vi "Set-Test-Clear Saved Tag.vi"(8 "op":enum16{"test", "clear", "set"}(ring), 11 "instVIref":T1) -> (0 "saved":bool, 3 "instVIref out":T1)   [LabVIEW 2020, in "NI_TargetHelper.lvlib"]
uses:
  <vilib>/TargetSupport/NI_TargetHelper/NI_TargetHelper.lvlib
  <vilib>/TargetSupport/NI_TargetHelper/Instance VIref.ctl
  <vilib>/UserTags/UserTags.lvlib
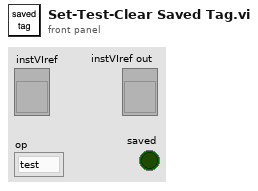
[diagram p1: front panel]
types:
  T1 = typedef "NI_TargetHelper.lvlib/Instance VIref.ctl" = refnum<vi>
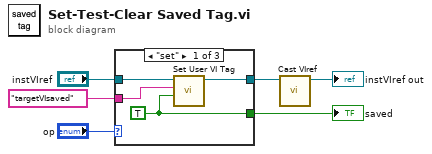
[diagram p0: block diagram]
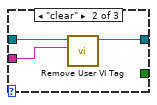
[diagram p2: hidden frame]
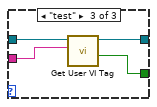
[diagram p3: hidden frame]
diagram:
  n1 = case shown="\"set\"" "op" {
    tunnel: "instVIref" -> [w10 w12 w17]
    tunnel: [w7 _ w14] -> w6
    tunnel: [w9 w11 w16] -> w3
    tunnel: "targetVIsaved" ("Tag Name") -> [w8 w13 w15]
    frame "set" {
      w7 = TRUE
      n2 = call <vilib>:"Set User VI Tag.vi"("Value"=w7, "Tag Name"=w8, "VI Refnum"=w10) -> ("dup VI Refnum"=w9:refnum<vi>)  [unwired: 6 in, 2 out]
    }
    frame "clear" {
      n3 = call <vilib>:"Remove User VI Tag.vi"("Tag Name"=w13, "Generic Refnum"=w12) -> ("dup Generic Refnum"=w11:refnum<vi>)  [unwired: 7 in, 2 out]
    }
    frame "test" {
      n4 = call <vilib>:"Get User VI Tag.vi"("Tag Name"=w15, "VI Refnum"=w17) -> ("Was Tag Found?"=w14:bool, "dup VI Refnum"=w16:refnum<vi>)  [unwired: 6 in, 2 out]
    }
  }
  "saved" <- w6
  n5 = call <vilib>:"Cast VIref.vi"("VI Refnum"=w3) -> ("instVIref"=→"instVIref out":T1)  [unwired: 10 in]
